vi "Filter Shared Variables by Type (Plot Data Clusters Only).vi"(8 "error in":errorcluster, 10 "Variable Descriptions":T1[](array[typedef]), 11 "Variable References":refnum<k21>[](array[refnum])) -> (0 "error out":errorcluster, 2 "Variable Descriptions":T1[](array[typedef]), 3 "Shared Variable References":refnum<k21>[](array[refnum]))   [LabVIEW 2017, in "DTacq Plot Display Library.lvlib"]
doc: "Filters arrays of variable references, and their descriptions, so that only plot data types are included."
uses:
  DTacq Plot Display Library.lvlib
  Network Shared Variables/Typedefs/Shared Variable Properties--Cluster.ctl
  Plot Data--Cluster.ctl
  Network Shared Variables/Typedefs/X and Y Variant Arrays--Cluster.ctl
  <resource>/objmgr/ni.var.rc
  Network Shared Variables/Shared Variables Library.lvlib
  <vilib>/Utility/Data Type/NI_Data Type.lvlib
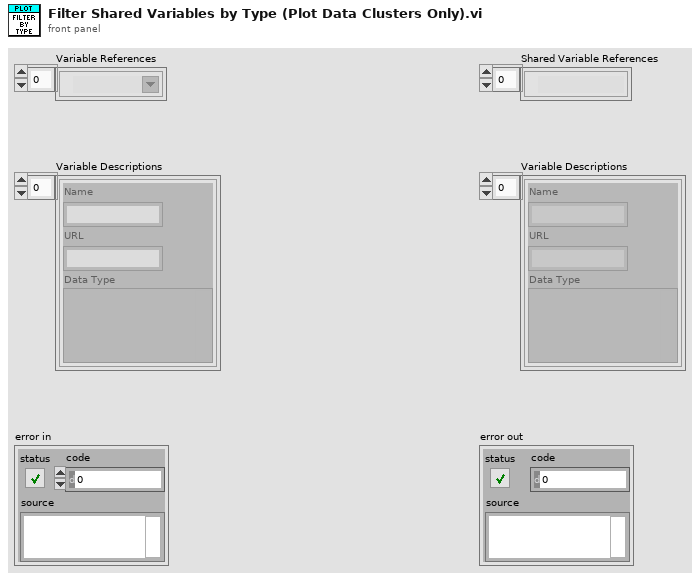
[diagram p1: front panel]
types:
  T1 = typedef "Shared Variables Library.lvlib/Shared Variable Properties--Cluster.ctl" = cluster{"Name":string, "URL":string, "Data Type":variant}
  T2 = typedef "DTacq Plot Display Library.lvlib/Plot Data--Cluster.ctl" = cluster{"Last Update":timestamp, "Data Cluster":T3}
  T3 = typedef "Shared Variables Library.lvlib/X and Y Variant Arrays--Cluster.ctl" = cluster{"X-Data":variant[], "Y-Data":variant[]}
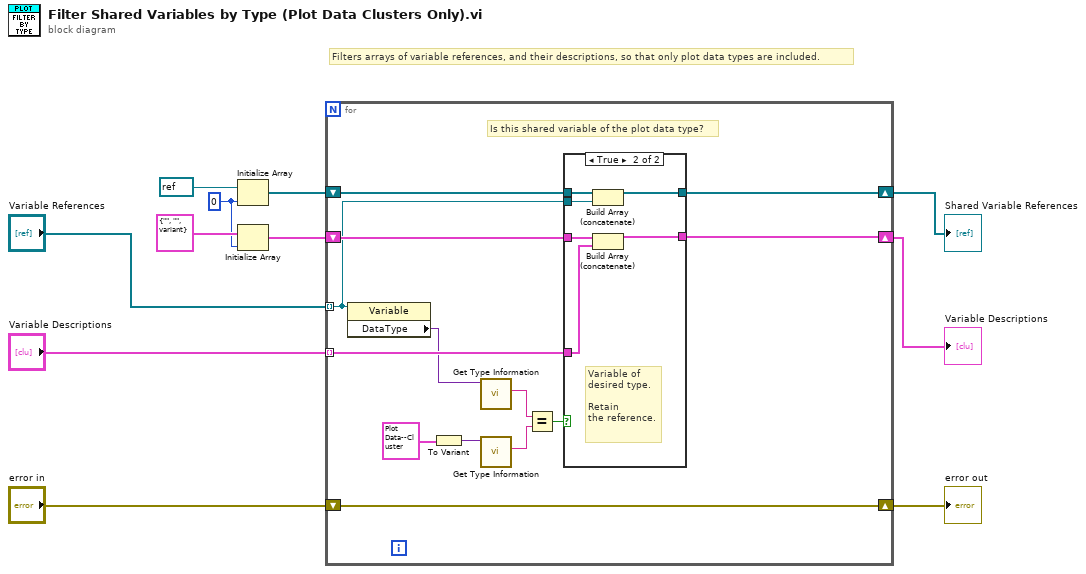
[diagram p0: block diagram]
diagram:
  w5 = 0 ("dimension size")
  # "Filters arrays of variable references, and their descriptions, so that only plot data types are included."
  n1 = Initialize Array(refnum<k21> refnum, w5) -> (w4:refnum<k21>[])
  n2 = Initialize Array(T1 {"Name"="", "URL"="", "Data Type"=variant} ("Shared Variable Data"), w5) -> (w3:T1[])
  n3 = for {
    tunnel: "Variable References" -> [w14] mode=indexing
    tunnel: "Variable Descriptions" -> [w17] mode=indexing
    shift-right: [w16] -> w11
    shift-left: "error in" -> [w16]
    shift-right: [w13] -> w2
    shift-left: w4 -> [w19]
    shift-right: [w12] -> w1
    shift-left: w3 -> [w18]
    # "Is this shared variable of the plot data type?"
    n4 = property class="Variable"(reference=w14) -> ("DataType"=w15:variant)  [unwired: 1 in, 2 out]
    n5 = To Variant(anything=T2 {"Last Update"=timestamp(0 s since 1904-01-01), "Data Cluster"={"X-Data"=[], "Y-Data"=[]}} ("Plot Data")) -> (Variant=w23:variant)
    n6 = call <vilib>:"Get Type Information.vi"("Variant"=w15) -> ("Name"=w21:string)  [unwired: 6 in, 4 out]
    n7 = call <vilib>:"Get Type Information.vi"("Variant"=w23) -> ("Name"=w22:string)  [unwired: 6 in, 4 out]
    n8 = Equal?(x=w21, y=w22) -> (x = y?=w20:bool)
    n9 = case shown="True" w20 {
      tunnel: w19 -> [w26 w32]
      tunnel: w18 -> [w25 w31]
      tunnel: w17 -> [_ w30]
      tunnel: w14 -> [_ w29]
      tunnel: [w26 w28] -> w13
      tunnel: [w25 w27] -> w12
      frame False {
        # "Variable of \nundesired type.\n\nDo not retain\nthe reference."
      }
      frame True {
        # "Variable of \ndesired type.\n\nRetain\nthe reference."
        n10 = Build Array (concatenate)(w32, w29) -> (w28:refnum<k21>[])
        n11 = Build Array (concatenate)(w31, w30) -> (w27:T1[])
      }
    }
  }
  "Shared Variable References" <- w2
  "Variable Descriptions" <- w1
  "error out" <- w11
